vi "HFRR ADV v019 new software.vi"() -> ()   [LabVIEW 2025] (continued)
          tunnel: [w1633 w1647] -> w1619
          tunnel: w1611 -> [w1632 w1651]
          frame No Error {
            n1452 = property class="Instr"(reference=w1632, error in=w1631) -> (reference out=w1629:refnum<visa-resource-name>, error out=w1630:errorcluster, "Serial Settings:Number of Bytes at Serial Port"=w1626:u32)
            n1453 = Greater?(x=w1626, y=u32 5) -> (0:w1625:bool)
            n1454 = Not(x=w1625) -> (.not. x?=→"Port 1a":bool)
            n1455 = while {
              tunnel: [w1642] -> w1633
              tunnel: [w1641] -> w1634
              tunnel: w1630 -> [w1640]
              tunnel: w1629 -> [w1639]
              stop <- TRUE stop-if-true
              n1456 = property class="Instr" props=["Serial Settings:Number of Bytes at Serial Port"](reference=w1639, error in=w1640) -> (reference out=w1644:refnum<visa-resource-name>, error out=w1643:errorcluster)  [unwired: 1 out]
              n1457 = VISA Read(VISA resource name=w1644, byte count=u32 50, error in (no error)=w1643) -> (VISA resource name out=w1641:refnum<visa-resource-name>, read buffer=→"UNI READ":string, error out=w1642:errorcluster)  [unwired: 1 out]
              n1458 = Wait (ms)(milliseconds to wait=u32 5) -> ()  [unwired: 1 out]
            }
          }
          frame Error {
            w1659 = u16 0 items=["None", "XON/XOFF", "RTS/CTS", "XON/XOFF & RTS/CTS", "DTR/DSR", "XON/XOFF & DTR/DSR"] ("flow control (0:none)  2")
            w1657 = u16 10 items=["1.0"=10, "1.5"=15, "2.0"=20] ("stop bits 2")
            w1655 = u16 0 items=["None", "Odd", "Even", "Mark", "Space"] ("parity 2")
            w1656 = u32 10000  # timeout (10sec)
            n1459 = VISA Close(VISA resource name=w1651, error in (no error)=w1649) -> (error out=w1652:errorcluster)
            n1460 = local write "Port 1a"(FALSE ("Port 1a")) -> ()
            n1461 = local read "Com Port 1"() -> (w1646:refnum<visa-resource-name>)
            n1462 = call <vilib>:"Clear Errors.vi"("error in (no error)"=w1652) -> ("error out"=w1650:errorcluster)  [unwired: 5 in, 1 out]
            n1463 = call-poly "VISA Configure Serial Port"("VISA resource name"=w1646, "timeout (10sec)"=w1656, "baud rate (9600)"=u32 250000 ("baud rate  2"), "data bits (8)"=u16 8 ("data bits  2"), "parity (0:none)"=w1655, "error in (no error)"=w1650, "stop bits (10: 1 bit)"=w1657, "flow control (0:none)"=w1659) -> ("VISA resource name out"=w1660:refnum<visa-resource-name>, "error out"=w1661:errorcluster)  [unwired: 6 in]
            n1464 = flat-sequence {
              tunnel: w1660 -> [w1663]
              tunnel: w1661 -> [w1662]
              tunnel: [w1663] -> w1653
              tunnel: [w1662] -> w1647
              frame #0 {
                n1465 = Wait (ms)(milliseconds to wait=u32 50) -> ()  [unwired: 1 out]
              }
            }
            "Residual Uno" <- ""
            "Port 1 Error" <- w1647
          }
        }
        n1466 = local read "Quit"() -> (w1608:bool)
        "Error Uno" <- w1613
      }
      n1467 = VISA Close(VISA resource name=w1606, error in (no error)=w1605) -> (error out=w1603:errorcluster)
      n1468 = call <vilib>:"Clear Errors.vi"("error in (no error)"=w1603) -> ()  [unwired: 5 in, 2 out]
    }
    frame Enabled {
    }
  }
  n1469 = while {
    stop <- w1674 stop-if-true
    # "V0OLTAGE TO STROKE (peice vise calibration)"
    n1470 = local read "LVDT MIN"() -> (w1665:dbl)
    n1471 = Wait (ms)(milliseconds to wait=u32 10) -> ()  [unwired: 1 out]
    n1472 = local read "LVDT Peak"() -> (w1666:dbl)
    n1473 = formula code="// Dynamic Parameterized Linear Interpolation Node\n// Inputs: vpp_val, voltages (Array), distances (Array)\n// Outputs: stroke\n\nint i = 0;\nint segments = 11; // 12 points make 11 interpolation segments\n\n// 1. Lower Boundary Clamp\nif (vpp_val <= voltages[0]) {\n    stroke = distances[0];\n}\n// 2. Upper Boundary Clamp\nelse if (vpp_val >= voltages[segments]) {\n    stroke = distances[segments];\n}\n// 3. Dynamic Segment Search Loop\nelse {\n    stroke = distances[0]; // Fallback baseline\n    for (i = 0; i < segments; i++) {\n        if (vpp_val >= voltages[i] && vpp_val <= voltages[i+1]) {\n            // Standard linear interpolation formula using array lookups\n            stroke = distances[i] + (vpp_val - voltages[i]) * (distances[i+1] - distances[i]) / (voltages[i+1] - voltages[i]);\n            break; // Segment found, safely exit the loop\n        }\n    }\n}"("vpp_val"=w1666, "voltages"="calibration values", "distances"="STROKE") -> ("stroke"=→"LVDT STROKE":dbl)
    n1474 = local read "Calibration Tare Value"() -> (w1670:dbl)
    n1475 = local read "Calibration Tare"() -> (w1668:bool)
    n1476 = Subtract(x=w1665, y=w1670) -> (x-y=→"LVDT STROKE  Calibration":dbl)
    n1477 = case shown="True" w1668 {
      selector: w1668 -> [_ w1676]
      tunnel: w1665 -> [_ w1677]
      frame False {
      }
      frame True {
        n1478 = Not(x=w1676) -> (.not. x?=w1675:bool)
        n1479 = local write "Calibration Tare"(w1675) -> ()
        "Calibration Tare Value" <- w1677
      }
    }
    n1480 = local read "Quit"() -> (w1674:bool)
  }
  n1481 = while {
    stop <- w1697 stop-if-true
    n1482 = call <vilib>:"High Resolution Polling Wait.vi"("seconds to wait"=0.02) -> ()  [unwired: 10 in, 1 out]
    n1483 = local read "Due read"() -> (w1695:string)
    n1484 = Spreadsheet String To Array(delimiter (Tab)=";", format string="", spreadsheet string=w1695, array type (2D Dbl)=string[] []) -> (array=w1692:string[])
    n1485 = Fract/Exp String To Number(string=w1692) -> (number=w1691:dbl[])  [unwired: 3 in, 1 out]
    n1486 = Index Array(array=w1691) -> (element #1=→"Sample Temperature":dbl, element #2=→"Target Sample Temperature":dbl, element #3=→"Current Duty Cycle":dbl, element #4=→"Ambient Temperature":dbl, element #5=→"Dac Status":dbl, element #6=→"Vpp":dbl, element #7=→"Active Error Code":dbl, element #8=→"Kp":dbl, element #9=→"Ki":dbl, element #10=→"Kd":dbl, element #11=→"SampleRaw":dbl, element #12=→"AmbRaw":dbl)  [unwired: 12 in]
    n1487 = local read "Quit"() -> (w1697:bool)
  }
  n1488 = while {
    shift-right: [w1711] -> w39
    shift-left: _ -> [w1702]
    shift-right: [w1710] -> w38
    shift-left: errorcluster {"status"=FALSE, "code"=0, "source"="Init"} ("error out") -> [w1704]
    tunnel: [w1699] -> w43
    tunnel: [w1709] -> _
    i -> [w1709]
    stop <- w1699 stop-if-true
    n1489 = local read "Com Port 2"() -> (w1703:refnum<visa-resource-name>)
    n1490 = local read "Port 2a"() -> (w1705:bool)
    n1491 = Unbundle(w1704) -> ("status"=→"Port 4":bool)  [unwired: 2 out]
    n1492 = call <vilib>:"High Resolution Polling Wait.vi"("seconds to wait"=0.02) -> ()  [unwired: 10 in, 1 out]
    n1493 = local read "Port 4"() -> (w1706:bool)
    n1494 = Not Equal?(x=w1703, y=w1702) -> (x != y?=w1701:bool)
    n1495 = Or(x=w1706, y=w1705) -> (x .or. y?=w1708:bool)
    n1496 = case shown="False" w1708 {
      frame False {
        w1714 = TRUE ("Visible")
        n1497 = property on="Port 2a" class="Bool (strict)"("Visible"=w1714) -> ()  [unwired: 2 in, 2 out]
        n1498 = property on="Port 4" class="Bool (strict)"("Visible"=w1714) -> ()  [unwired: 2 in, 2 out]
      }
      frame True {
        w1715 = TRUE ("Visible")
        n1499 = property on="Port 2a" class="Bool (strict)"("Visible"=w1715) -> ()  [unwired: 2 in, 2 out]
        n1500 = property on="Port 4" class="Bool (strict)"("Visible"=w1715) -> ()  [unwired: 2 in, 2 out]
      }
    }
    n1501 = case shown="True" w1701 {
      tunnel: [w1712 errorcluster {"status"=TRUE, "code"=0, "source"="Init"} ("error out")] -> w1700
      tunnel: w1704 -> [w1712 _]
      frame False {
      }
      frame True {
      }
    }
    n1502 = case shown="No Error" w1700 {
      selector: w1700 -> [w1728 w1759]
      tunnel: [w1721 w1764] -> w1711
      tunnel: [w1729 w1757] -> w1710
      tunnel: w1702 -> [w1730 w1762]
      frame No Error {
        n1503 = property class="Instr" props=["Serial Settings:Number of Bytes at Serial Port"](reference=w1730, error in=w1728) -> (reference out=w1722:refnum<visa-resource-name>, error out=w1727:errorcluster)  [unwired: 1 out]
        n1504 = while {
          tunnel: [w1738] -> w1723
          tunnel: [w1737] -> w1724
          tunnel: w1727 -> [w1736]
          tunnel: w1722 -> [w1735]
          tunnel: [w1734] -> _
          i -> [w1734]
          stop <- TRUE stop-if-true
          n1505 = property class="Instr" props=["Serial Settings:Number of Bytes at Serial Port"](reference=w1735, error in=w1736) -> (reference out=w1740:refnum<visa-resource-name>, error out=w1739:errorcluster)  [unwired: 1 out]
          n1506 = VISA Read(VISA resource name=w1740, byte count=u32 1000, error in (no error)=w1739) -> (VISA resource name out=w1737:refnum<visa-resource-name>, read buffer=→"Due read":string, error out=w1738:errorcluster)  [unwired: 1 out]
        }
        n1507 = local read "Command"() -> (w1720:string)
        n1508 = call <vilib>:"Trim Whitespace.vi"("string"=w1720) -> ("trimmed string"=w1719:string)  [unwired: 1 in]
        n1509 = Not Equal?(x=w1719, y="") -> (x != y?=w1725:bool)
        n1510 = VISA Flush I/O Buffer(VISA resource name=w1724) -> (VISA resource name out=w1717:refnum<visa-resource-name>, error out=→"error out 10":errorcluster)  [unwired: 2 in]
        n1511 = case shown="True" w1725 {
          tunnel: w1717 -> [w1742 w1747]
          tunnel: [w1742 w1751] -> w1721
          tunnel: w1723 -> [w1741 w1746]
          tunnel: [w1741 w1749] -> w1729
          tunnel: w1719 -> [_ w1745]
          tunnel: [_ w1748] -> _
          frame False {
            # "DATA  WRITE LOOP"
          }
          frame True {
            n1512 = Concatenate Strings(w1745, "\r\n") -> (w1744:string)
            n1513 = VISA Write(VISA resource name=w1747, write buffer=w1744, error in (no error)=w1746) -> (VISA resource name out=w1751:refnum<visa-resource-name>, return count=w1748:u32, error out=w1750:errorcluster)
            n1514 = flat-sequence {
              tunnel: w1750 -> [w1753]
              tunnel: [w1753] -> w1749
              frame #0 {
                n1515 = local write "Command"("" ("Command")) -> ()
                n1516 = Wait (ms)(milliseconds to wait=u32 5) -> ()  [unwired: 1 out]
              }
            }
          }
        }
        "Port 2a" <- TRUE ("Port 2a")
      }
      frame Error {
        w1770 = u16 0 items=["None", "XON/XOFF", "RTS/CTS", "XON/XOFF & RTS/CTS", "DTR/DSR", "XON/XOFF & DTR/DSR"] ("flow control (0:none)  2")
        w1768 = u16 10 items=["1.0"=10, "1.5"=15, "2.0"=20] ("stop bits 2")
        w1766 = u16 0 items=["None", "Odd", "Even", "Mark", "Space"] ("parity 2")
        w1767 = u32 10000  # timeout (10sec)
        n1517 = VISA Clear(VISA resource name=w1762, error in (no error)=w1759) -> (VISA resource name out=w1761:refnum<visa-resource-name>, error out=w1760:errorcluster)
        n1518 = VISA Close(VISA resource name=w1761, error in (no error)=w1760) -> (error out=w1763:errorcluster)
        n1519 = call <vilib>:"Clear Errors.vi"("error in (no error)"=w1763) -> ()  [unwired: 5 in, 2 out]
        n1520 = local write "Port 2a"(FALSE ("Port 2a")) -> ()
        n1521 = local read "Com Port 2"() -> (w1756:refnum<visa-resource-name>)
        "visa due" <- w1756
        n1522 = call-poly "VISA Configure Serial Port"("VISA resource name"=w1756, "timeout (10sec)"=w1767, "baud rate (9600)"=u32 250000 ("baud rate  2"), "data bits (8)"=u16 8 ("data bits  2"), "parity (0:none)"=w1766, "stop bits (10: 1 bit)"=w1768, "flow control (0:none)"=w1770) -> ("VISA resource name out"=w1771:refnum<visa-resource-name>, "error out"=w1772:errorcluster)  [unwired: 7 in]
        n1523 = flat-sequence {
          tunnel: w1771 -> [w1774]
          tunnel: w1772 -> [w1773]
          tunnel: [w1774] -> w1764
          tunnel: [w1773] -> w1757
          frame #0 {
            n1524 = Wait (ms)(milliseconds to wait=u32 50) -> ()  [unwired: 1 out]
          }
        }
        "Residual Due" <- ""
        "Port 2 Error" <- w1757
      }
    }
    n1525 = local read "Quit"() -> (w1699:bool)
    "Error Due" <- w1704
  }
  n1526 = local write "FRICVALZ"(0.0 ("FRICVALZ")) -> ()
  n1527 = property on="RUN" class="Bool (strict)"("Visible"=TRUE) -> ()  [unwired: 2 in, 2 out]
  n1528 = while {
    tunnel: [w1791] -> _
    tunnel: [w1776] -> w53
    i -> [w1791]
    stop <- w1776 stop-if-true
    n1529 = local read "conststatus"() -> (w1780:dbl)
    n1530 = local read "Main Tab"() -> (w1778:T2)
    n1531 = local read "EDIT"() -> (w1797:bool)
    n1532 = local read "Rate"() -> (w1796:dbl)
    n1533 = case shown="True" w1797 {
      tunnel: [FALSE TRUE] -> w1783
      frame False {
      }
      frame True {
      }
    }
    n1534 = property on="Time slide" class="Slide (strict)"("Scale.Range:Maximum"=2500.0) -> ()  [unwired: 2 in, 2 out]
    n1535 = Equal?(x=w1778, y=T27."About" ("Main Tab")) -> (x = y?=w1789:bool)
    n1536 = Equal?(x=w1780, y=0.0) -> (x = y?=w1781:bool)
    n1537 = Divide(x=1.0, y=w1796) -> (x/y=w1792:dbl)
    "Time 2" <- w1792
    n1538 = case shown="True" w1781 {
      frame False {
      }
      frame True {
        # "C:\\WinDucom\\calibrate WO 2391.dcf"
        n1539 = local write "Lan flag"(22) -> ()
        n1540 = local write "conststatus"(10.0 ("rpm value : 2")) -> ()
        n1541 = String To Path(string="C:\\LAB-IQ\\calibrate WO 2465.dcf") -> (path=w1803:path)
        n1542 = Open/Create/Replace File "Open File"(file path (use dialog)=w1803) -> (refnum out=w1801:refnum<file>)  [unwired: 5 in, 2 out]
        n1543 = for {
          N: 23 -> [_]
          tunnel: w1801 -> [w1812]
          i -> [w1806]
          (unwired) TRUE ("line mode (F)")
          n1544 = Read from Text File "Read File"(file (use dialog)=w1812) -> (text=w1811:string)  [unwired: 3 in, 3 out]
          n1545 = Match Pattern(string=w1811, regular expression="]") -> (after substring=w1809:string)  [unwired: 1 in, 3 out]
          n1546 = String Subset(string=w1811, offset (0)=5, length (rest)=10 ("length (rest)")) -> (substring=w1804:string)
          n1547 = Fract/Exp String To Number(string=w1804) -> (number=w1805:dbl)  [unwired: 3 in, 1 out]
          n1548 = Match Pattern(string=w1809, regular expression="-") -> (before substring=w1807:string)  [unwired: 1 in, 3 out]
          n1549 = case shown="4" w1806 {
            tunnel: w1805 -> [w1815 w1816 w1817 w1818 _ _ _ w1823 w1824 _ w1825 w1826 w1827 w1828 w1829 w1830 _ w1831 w1832 _ _ _ _ _]
            tunnel: w1807 -> [_ _ _ _ w1819 w1820 w1821 _ _ _ _ _ _ _ _ _ _ _ _ w1833 w1834 w1835 w1836 _]
            frame 0 {
              n1550 = local write "FRIC. FORCE :"(w1815) -> ()
            }
            frame 1 {
              n1551 = local write "TEMPERATURE :"(w1816) -> ()
            }
            frame 2 {
              n1552 = local write "HUMIDITY:"(w1817) -> ()
            }
            frame 3 {
              n1553 = local write "AIR TEMPERATURE :"(w1818) -> ()
            }
            frame 4 {
              n1554 = local write "Com Port 1"(w1819) -> ()
            }
            frame 5 {
              n1555 = local write "Com Port 2"(w1820) -> ()
              n1556 = local write "visa due"(w1820) -> ()
            }
            frame 6 {
              n1557 = String To Path(string=w1821) -> (path=w1822:path)
              n1558 = local write "File Path"(w1822) -> ()
              "String" <- w1821
            }
            frame 7 {
              n1559 = local write "DISPLACEMENT :"(w1823) -> ()
            }
            frame 8 {
              n1560 = local write "STROKE GAIN :"(w1824) -> ()
            }
            frame 9 {
            }
            frame 10 {
              n1561 = local write "Language Selection"(w1825) -> ()
            }
            frame 11 {
              n1562 = local write "CH-POWER +"(w1826) -> ()
            }
            frame 12 {
              n1563 = local write "CH-POWER -"(w1827) -> ()
            }
            frame 13 {
              n1564 = local write "CH-HEATER"(w1828) -> ()
            }
            frame 14 {
              n1565 = local write "CH-HUMIDITY WET"(w1829) -> ()
            }
            frame 15 {
              n1566 = local write "CH-HUMIDITY DRY"(w1830) -> ()
            }
            frame 16 {
            }
            frame 17 {
              n1567 = local write "AIR TEMP INTERCEPT:"(w1831) -> ()
            }
            frame 18 {
              n1568 = local write "TEMP INTERCEPT:"(w1832) -> ()
            }
            frame 21 {
              n1569 = local write "S.NO"(w1833) -> ()
            }
            frame 22 {
              n1570 = local write "Com Port 3"(w1834) -> ()
            }
            frame 20 {
              n1571 = local write "Camera Port :"(w1835) -> ()
            }
            frame 19 {
              n1572 = local write "C3 :"(w1836) -> ()
            }
            frame 23, Default {
            }
          }
        }
      }
    }
    n1573 = Select(t=u32 2500 ("milliseconds to wait"), s=w1789, f=u32 500 ("milliseconds to wait")) -> (s? t:f=w1787:u32)
    n1574 = Multiply(x=w1792, y=w1787) -> (x*y=w1794:dbl)
    n1575 = property on="Time slide" class="Slide (strict)"("Visible"=w1783) -> ()  [unwired: 2 in, 2 out]
    n1576 = call "Elapsed Time2"("Time Target (s)"=w1794, "Auto Reset"=TRUE) -> ("Time has Elapsed"=w1784:bool)  [unwired: 10 in, 7 out]
    n1577 = case shown="True" w1784 {
      frame False {
      }
      frame True {
        n1578 = stacked-sequence {
          frame #0 {
            # "DATA PROCESSING"
            # "115 mV/N"
            n1579 = local read "Sample Temperature"() -> (w1839:dbl)
            n1580 = local read "RH Numeric:"() -> (w1846:dbl)
            n1581 = local read "HUMIDITY:"() -> (w1847:dbl)
            n1582 = local read "FRICVALZ"() -> (w1858:dbl)
            n1583 = local read "Friction"() -> (w1842:dbl)
            n1584 = Multiply(x=w1846, y=w1847) -> (x*y=→"Humidity ( %RH )" →"Hum" →"Hum 2":dbl)
            n1585 = call <vilib>:"Mean PtByPt.vi"("x"=w1839, "sample length"=100) -> ("mean"=w1838:dbl)  [unwired: 2 in, 1 out]
            "TEMP 2" <- w1838
            "TEMP 3" <- w1838
            n1586 = Subtract(x=w1842, y=w1858) -> (x-y=w1853:dbl)
            "FF 2" <- w1853
            "FF 4" <- w1853
            n1587 = local read "Ambient Temperature"() -> (→"AIR TEMP":dbl)
            n1588 = local read "TEMP"() -> (w1857:dbl)
            n1589 = local write "FF 3"(w1853) -> ()
            n1590 = Compound Arithmetic op=OR("FRICVALZ 4", "FRICVALZ 3", "FRICVALZ 2") -> (w1849:bool)
            n1591 = case shown="True" w1849 {
              tunnel: w1842 -> [_ w1864]
              frame False {
              }
              frame True {
                w1863 = FALSE ("FRICVALZ")
                n1592 = local write "FRICVALZ 3"(w1863) -> ()
                n1593 = local write "FRICVALZ 2"(w1863) -> ()
                n1594 = local write "FRICVALZ 4"(w1863) -> ()
                "FRICVALZ" <- w1864
              }
            }
            n1595 = Not A Number/Path/Refnum?(number/path/refnum=w1857) -> (NaN/Path/Refnum?=w1856:bool)
            n1596 = Not A Number/Path/Refnum?(number/path/refnum=w1853) -> (NaN/Path/Refnum?=w1855:bool)
            n1597 = Divide(x=w1853, y=1.96) -> (x/y=w1850:dbl)
            n1598 = Compound Arithmetic op=OR(w1856, w1855) -> (w1854:bool)
            n1599 = Not A Number/Path/Refnum?(number/path/refnum=w1850) -> (NaN/Path/Refnum?=w1851:bool)
            n1600 = case shown="True" w1854 {
              frame False {
              }
              frame True {
                n1601 = local write "TEMP"(0.0 ("TEMP")) -> ()
                n1602 = local write "FF 2"(0.0 ("FF 2")) -> ()
                n1603 = local write "reinit"(TRUE ("reinit")) -> ()
              }
            }
            n1604 = local write "TEMP"(w1838) -> ()
            n1605 = Select(t=0.0, s=w1851, f=w1850) -> (s? t:f=w1841:dbl)
            "COF 2" <- w1841
            n1606 = local write "COF 3"(w1841) -> ()
          }
        }
      }
    }
    n1607 = Wait (ms)(milliseconds to wait=u32 50) -> ()  [unwired: 1 out]
    n1608 = local read "Quit"() -> (w1776:bool)
    "Rate" <- 2500.0 ("No of Samples")
  }
  n1609 = while {
    tunnel: w56 -> [_]
    tunnel: [w1891] -> _
    tunnel: [w1867] -> w55
    i -> [w1891]
    stop <- w1867 stop-if-true
    # "C:\\LAB-IQ-NXT\\Scar View.exe"
    n1610 = local read "OK Button 16"() -> (w1880:bool)
    n1611 = local read "Main Tab"() -> (w1873:T2)
    n1612 = local read "service 3"() -> (w1874:bool)
    n1613 = local read "OPEN 6"() -> (w1876:bool)
    n1614 = local read "EDIT 2"() -> (w1878:bool)
    n1615 = flat-sequence {
      frame #0 {
        n1616 = local read "SAVE 2"() -> (w2493:bool)
        n1617 = stacked-sequence {
          frame #0 {
            n1618 = local read "EDIT"() -> (w2547:bool)
            n1619 = case shown="True" w2547 {
              tunnel: [u8 2 ("Disabled") u8 0 ("Disabled")] -> _
              frame False {
                w2549 = FALSE
                n1620 = local write "Password"("") -> ()
                n1621 = property on="SrvM CP" class="Bool (strict)"("Visible"=w2549) -> ()  [unwired: 2 in, 2 out]
                n1622 = property on="message" class="Str"("Visible"=w2549) -> ()  [unwired: 2 in, 2 out]
                n1623 = local write "x = y?"(w2549) -> ()
                n1624 = property on="Password" class="Str"("Visible"=w2549) -> ()  [unwired: 2 in, 2 out]
                n1625 = property on="ENTER THE NEW PASSWORD" class="Str"("Visible"=w2549) -> ()  [unwired: 2 in, 2 out]
                n1626 = property on="ENTER CURRENT PASSWORD" class="Str"("Visible"=w2549) -> ()  [unwired: 2 in, 2 out]
                n1627 = local write "SrvM CP"(w2549) -> ()
              }
              frame True {
                w2552 = TRUE
                n1628 = property on="SrvM CP" class="Bool (strict)"("Visible"=w2552) -> ()  [unwired: 2 in, 2 out]
                n1629 = property on="Password" class="Str"("Visible"=w2552) -> ()  [unwired: 2 in, 2 out]
              }
            }
            "dipl pwd" <- "@143$\n" ("dipl pwd")
          }
          frame #1 {
            # "Gain password"
            n1630 = String To Byte Array(string="ENTER CURRENT PASSWORD") -> (unsigned byte array=w2557:u8[])
            n1631 = Search 1D Array(1D array=w2557, element=u8 10) -> (index of element=w2560:i32)  [unwired: 1 in]
            n1632 = Index Array(array=w2557, index=w2560) -> (element=w2556:u8)
            n1633 = Equal?(x=w2556, y=10) -> (x = y?=w2554:bool)
            n1634 = case shown="True" w2554 {
              frame False {
                n1635 = property on="ENTER THE NEW PASSWORD" class="Str"("Visible"=FALSE) -> ()  [unwired: 2 in, 2 out]
              }
              frame True {
                # "password"
                # "change password logic"
                n1636 = local read "ENTER CURRENT PASSWORD"() -> (w2573:string)
                n1637 = local read "dipl pwd"() -> (w2567:string)
                n1638 = String To Byte Array(string=w2573) -> (unsigned byte array=w2575:u8[])
                n1639 = String To Byte Array(string=w2567) -> (unsigned byte array=w2568:u8[])
                n1640 = Array Size(array=w2575) -> (size(s)=w2572:i32)
                n1641 = Array Size(array=w2568) -> (size(s)=w2570:i32)
                n1642 = for {
                  N: w2572 -> [_]
                  tunnel: w2575 -> [w2599]
                  tunnel: [w2597] -> w2576 mode=indexing
                  tunnel: w2572 -> [w2591]
                  i -> [w2592]
                  n1643 = Decrement(x=w2591) -> (x-1=w2589:i32)
                  n1644 = Equal?(x=w2592, y=w2589) -> (x = y?=w2590:bool)
                  n1645 = Index Array(array=w2599, index=w2592) -> (element=w2593:u8)
                  n1646 = Number To Decimal String(number=w2593) -> (decimal integer string=w2598:string)  [unwired: 1 in]
                  n1647 = Select(t="", s=w2590, f="\r") -> (s? t:f=w2595:string)
                  n1648 = Concatenate Strings(w2598, w2595) -> (w2597:string)
                }
                n1649 = for {
                  N: w2570 -> [_]
                  tunnel: w2568 -> [w2587]
                  tunnel: [w2585] -> w2569 mode=indexing
                  tunnel: w2570 -> [w2582]
                  i -> [w2583]
                  n1650 = Decrement(x=w2582) -> (x-1=w2581:i32)
                  n1651 = Equal?(x=w2583, y=w2581) -> (x = y?=w2580:bool)
                  n1652 = Index Array(array=w2587, index=w2583) -> (element=w2586:u8)
                  n1653 = Number To Decimal String(number=w2586) -> (decimal integer string=w2584:string)  [unwired: 1 in]
                  n1654 = Select(t="", s=w2580, f="\r") -> (s? t:f=w2577:string)
                  n1655 = Concatenate Strings(w2584, w2577) -> (w2585:string)
                }
                n1656 = local read "string"() -> (w2574:string)
                n1657 = Concatenate Strings(w2569) -> (w2563:string)
                n1658 = Concatenate Strings(w2574) -> (w2571:string)
                n1659 = Concatenate Strings(w2576) -> (w2564:string)
                n1660 = Equal?(x=w2564, y=w2571) -> (x = y?=w2566:bool)
                n1661 = Equal?(x=w2564, y=w2563) -> (x = y?=w2562:bool)
                n1662 = Or(x=w2566, y=w2562) -> (x .or. y?=w2565:bool)
                n1663 = case shown="True" w2565 {
                  frame False {
                  }
                  frame True {
                    n1664 = property on="ENTER THE NEW PASSWORD" class="Str"("Visible"=TRUE) -> ()  [unwired: 2 in, 2 out]
                  }
                }
              }
            }
          }
          frame #2 {
            n1665 = String To Byte Array(string="ENTER THE NEW PASSWORD") -> (unsigned byte array=w2602:u8[])
            n1666 = Search 1D Array(1D array=w2602, element=u8 10) -> (index of element=w2606:i32)  [unwired: 1 in]
            n1667 = Index Array(array=w2602, index=w2606) -> (element=w2604:u8)
            n1668 = Equal?(x=w2604, y=10) -> (x = y?=w2601:bool)
            n1669 = case shown="False" w2601 {
              frame False {
              }
              frame True {
                n1670 = local write "EDIT"(FALSE) -> ()
                n1671 = local write "SrvM CP"(FALSE) -> ()
                n1672 = local read "ENTER THE NEW PASSWORD"() -> (w2609:string)
                n1673 = String To Byte Array(string=w2609) -> (unsigned byte array=w2614:u8[])
                n1674 = Array Size(array=w2614) -> (size(s)=w2611:i32)
                n1675 = for {
                  N: w2611 -> [_]
                  tunnel: w2614 -> [w2627]
                  tunnel: [w2624] -> w2616 mode=indexing
                  tunnel: w2611 -> [w2619]
                  i -> [w2617]
                  n1676 = Decrement(x=w2619) -> (x-1=w2620:i32)
                  n1677 = Equal?(x=w2617, y=w2620) -> (x = y?=w2621:bool)
                  n1678 = Index Array(array=w2627, index=w2617) -> (element=w2626:u8)
                  n1679 = Number To Decimal String(number=w2626) -> (decimal integer string=w2625:string)  [unwired: 1 in]
                  n1680 = Select(t="", s=w2621, f="\r") -> (s? t:f=w2618:string)
                  n1681 = Concatenate Strings(w2625, w2618) -> (w2624:string)
                }
                n1682 = local read "file path"() -> (w2608:path)
                n1683 = Concatenate Strings(w2616) -> (w2610:string)
                n1684 = Delete(path (use dialog)=w2608) -> (deleted path=w2612:path)  [unwired: 4 in, 2 out]
                n1685 = call <vilib>:"Write Characters To File.vi"("append to file? (new file:F)"=FALSE, "character string"=w2610, "file path (dialog if empty)"=w2612) -> ()  [unwired: 2 in, 1 out]
              }
            }
          }
          frame #3 {
            n1686 = case shown="True" "SrvM CP" {
              frame False {
                w2630 = ""
                n1687 = local write "ENTER CURRENT PASSWORD"(w2630) -> ()
                n1688 = local write "ENTER THE NEW PASSWORD"(w2630) -> ()
                n1689 = property on="ENTER CURRENT PASSWORD" class="Str"("Visible"=FALSE) -> ()  [unwired: 2 in, 2 out]
              }
              frame True {
                n1690 = property on="ENTER THE NEW PASSWORD" class="Str"() -> ("Visible"=w2631:bool)  [unwired: 2 in, 2 out]
                n1691 = Not(x=w2631) -> (.not. x?=w2632:bool)
                n1692 = property on="ENTER CURRENT PASSWORD" class="Str"("Visible"=w2632) -> ()  [unwired: 2 in, 2 out]
              }
            }
          }
          frame #4 {
            n1693 = String To Byte Array(string="Password") -> (unsigned byte array=w2639:u8[])
            n1694 = Search 1D Array(1D array=w2639, element=u8 10) -> (index of element=w2637:i32)  [unwired: 1 in]
            n1695 = Index Array(array=w2639, index=w2637) -> (element=w2638:u8)
            n1696 = Equal?(x=w2638, y=10) -> (x = y?=w2634:bool)
            n1697 = case shown="True" w2634 {
              frame False {
              }
              frame True {
                # "password"
                # "password"
                n1698 = local read "Password"() -> (w2652:string)
                n1699 = String To Byte Array(string=w2652) -> (unsigned byte array=w2655:u8[])
                n1700 = String To Byte Array(string="@143$\n") -> (unsigned byte array=w2641:u8[])
                n1701 = Array Size(array=w2655) -> (size(s)=w2650:i32)
                n1702 = Array Size(array=w2641) -> (size(s)=w2646:i32)
                n1703 = for {
                  N: w2650 -> [_]
                  tunnel: w2655 -> [w2689]
                  tunnel: [w2687] -> w2656 mode=indexing
                  tunnel: w2650 -> [w2684]
                  i -> [w2685]
                  n1704 = Decrement(x=w2684) -> (x-1=w2683:i32)
                  n1705 = Index Array(array=w2689, index=w2685) -> (element=w2688:u8)
                  n1706 = Equal?(x=w2685, y=w2683) -> (x = y?=w2682:bool)
                  n1707 = Number To Decimal String(number=w2688) -> (decimal integer string=w2686:string)  [unwired: 1 in]
                  n1708 = Select(t="", s=w2682, f="\r") -> (s? t:f=w2679:string)
                  n1709 = Concatenate Strings(w2686, w2679) -> (w2687:string)
                }
                n1710 = for {
                  N: w2646 -> [_]
                  tunnel: w2641 -> [w2700]
                  tunnel: [w2698] -> w2644 mode=indexing
                  tunnel: w2646 -> [w2695]
                  i -> [w2696]
                  n1711 = Decrement(x=w2695) -> (x-1=w2694:i32)
                  n1712 = Index Array(array=w2700, index=w2696) -> (element=w2699:u8)
                  n1713 = Equal?(x=w2696, y=w2694) -> (x = y?=w2693:bool)
                  n1714 = Number To Decimal String(number=w2699) -> (decimal integer string=w2697:string)  [unwired: 1 in]
                  n1715 = Select(t="", s=w2693, f="\r") -> (s? t:f=w2690:string)
                  n1716 = Concatenate Strings(w2697, w2690) -> (w2698:string)
                }
                n1717 = local read "file path"() -> (w2640:path)
                n1718 = call <vilib>:"Read Characters From File.vi"("file path (dialog if empty)"=w2640) -> ("character string"=w2654:string)  [unwired: 5 in, 3 out]
                "string" <- w2654
                n1719 = flat-sequence {
                  tunnel: [w2657] -> w2651
                  frame #0 {
                    w2657 = ""
                    n1720 = local write "Password"(w2657) -> ()
                  }
                }
                n1721 = Concatenate Strings(w2644) -> (w2645:string)
                n1722 = Concatenate Strings(w2654) -> (w2653:string)
                n1723 = Concatenate Strings(w2656) -> (w2648:string)
                n1724 = Equal?(x=w2648, y=w2653) -> (x = y?=w2643:bool)
                n1725 = Equal?(x=w2648, y=w2645) -> (x = y?=w2649:bool)
                n1726 = Or(x=w2643, y=w2649) -> (x .or. y?=w2642:bool)
                "x = y?" <- w2642
                n1727 = case shown="True" w2642 {
                  selector: w2642 -> [w2659 _]
                  tunnel: w2651 -> [_ _]
                  frame False {
                    n1728 = And(x=w2659, y=TRUE ("Visible")) -> (x .and. y?=w2660:bool)
                    n1729 = property on="message" class="Str"("Visible"=w2660) -> ()  [unwired: 2 in, 2 out]
                  }
                  frame True {
                    n1730 = control-ref of="This VI"() -> (w2671:refnum<vi>)
                    n1731 = property class="VI"(reference=w2671) -> (reference out=w2662:refnum<vi>, error out=w2666:errorcluster, "Panel"=w2670:refnum<vi>)  [unwired: 1 in]
                    n1732 = property on="message" class="Str"("Visible"=FALSE) -> ()  [unwired: 2 in, 2 out]
                    n1733 = property class="Pnl"(reference=w2670, error in=w2666) -> (reference out=w2664:refnum<vi>, error out=w2667:errorcluster, "Panes[]"=w2669:refnum<vi>[])
                    n1734 = for {
                      tunnel: w2669 -> [w2678] mode=indexing
                      tunnel: T21."Always On" ("Horizontal Scrollbar Visibility") -> [w2677]
                      tunnel: w2667 -> [w2674]
                      tunnel: [w2673] -> w2665
                      n1735 = property class="Pane"(reference=w2678, error in=w2674, "HorizScrollbarVisibility"=w2677) -> (reference out=w2675:refnum<vi>, error out=w2676:errorcluster)
                      n1736 = Close Reference(reference=w2675, error in (no error)=w2676) -> (error out=w2673:errorcluster)
                    }
                    n1737 = Close Reference(reference=w2664, error in (no error)=w2665) -> (error out=w2663:errorcluster)
                    n1738 = Close Reference(reference=w2662, error in (no error)=w2663) -> (error out=→"error out 6":errorcluster)
                  }
                }
              }
            }
          }
        }
        n1739 = local read "x = y?"() -> (w2499:bool)
        n1740 = local read "HUMIDITY: 2"() -> (w2501:dbl)
        n1741 = local read "HUMIDITY:"() -> (w2500:dbl)
        n1742 = property on="Port 2 Error" class="Clust (strict)"("Visible"="EDIT") -> ()  [unwired: 2 in, 2 out]
        n1743 = property on="Port 1 Error" class="Clust (strict)"("Visible"="EDIT") -> ()  [unwired: 2 in, 2 out]
        n1744 = case shown="True" "SrvM CP 2" {
          frame False {
          }
          frame True {
            n1745 = local write "SrvM CP 2"(FALSE ("SrvM CP 2")) -> ()
            n1746 = local read "HUMIDITY: 2"() -> (w2540:dbl)
            n1747 = local read "TEMP INTERCEPT: 2"() -> (w2539:dbl)
            n1748 = local read "DISPLACEMENT : 4"() -> (w2543:dbl)
            n1749 = local read "TEMPERATURE : 2"() -> (w2542:dbl)
            n1750 = local read "STROKE GAIN : 2"() -> (w2544:dbl)
            n1751 = local read "FRIC. FORCE : 2"() -> (w2545:dbl)
            n1752 = local read "AIR TEMP INTERCEPT: 2"() -> (w2538:dbl)
            n1753 = local read "AIR TEMPERATURE : 2"() -> (w2541:dbl)
            n1754 = local write "HUMIDITY:"(w2540) -> ()
            n1755 = local write "AIR TEMP INTERCEPT:"(w2539) -> ()
            n1756 = local write "TEMPERATURE :"(w2542) -> ()
            n1757 = local write "FRIC. FORCE :"(w2545) -> ()
            n1758 = local write "STROKE GAIN :"(w2544) -> ()
            n1759 = local write "DISPLACEMENT :"(w2543) -> ()
            n1760 = local write "AIR TEMPERATURE :"(w2541) -> ()
            n1761 = local write "TEMP INTERCEPT:"(w2538) -> ()
          }
        }
        n1762 = Or(x="SAVE", y=w2493) -> (x .or. y?=w2494:bool)
        n1763 = And(x="EDIT", y=w2499) -> (x .and. y?=w2497:bool)
        n1764 = local read "DISPLACEMENT : 4"() -> (w2510:dbl)
        n1765 = local read "TEMPERATURE : 2"() -> (w2508:dbl)
        n1766 = local read "STROKE GAIN : 2"() -> (w2514:dbl)
        n1767 = local read "DISPLACEMENT :"() -> (w2509:dbl)
        n1768 = local read "FRIC. FORCE : 2"() -> (w2517:dbl)
        n1769 = local read "TEMPERATURE :"() -> (w2506:dbl)
        n1770 = local read "STROKE GAIN :"() -> (w2513:dbl)
        n1771 = local read "FRIC. FORCE :"() -> (w2516:dbl)
        n1772 = case shown="True" w2497 {
          tunnel: [u8 2 ("Disabled") u8 0 ("Disabled")] -> w2496
          tunnel: [w2861 TRUE ("Visible")] -> w2495
          frame False {
            w2861 = FALSE ("Visible")
            n1773 = local write "EDIT 2"(w2861) -> ()
          }
          frame True {
          }
        }
        n1774 = case shown="True" w2494 {
          frame False {
          }
          frame True {
            n1775 = stacked-sequence {
              seq-local: [w2709 _ _] -> [_ w2856 _]
              frame #0 {
                (unwired) i16 5 ("precision (6)")
                # "[CH1]    - FF\n[CH2]   - TEMPERATURE\n[CH3]    - Humidity\n[CH4]    - AIR TEMP\n[CH5]\\- Visa Uno\n[CH6] \\- Visa Due\n[CH7]  \\- file path\n[CH8]   - Displacement Gain\n[CHA]   - Stroke Gain\n[CHB]   - Stroke PID Gain\n[CHC]   -Language Selection\n[CHD]   -Power +\n[CHE]   -Power_\n[CHF]   -Heater\n[CHG]   -Humidity Wet\n[CHH]   -Humidity Dry\n[CHI]   -Integral Time"
                n1776 = local read "Language Selection"() -> (w2757:enum16{"English", "Russian"})
                n1777 = local read "CH-HUMIDITY WET"() -> (w2715:u16)
                n1778 = local read "CH-HUMIDITY DRY"() -> (w2712:u16)
                n1779 = local read "STROKE GAIN :"() -> (w2701:dbl)
                n1780 = local read "CH-POWER +"() -> (w2724:u16)
                n1781 = local read "CH-POWER -"() -> (w2721:u16)
                n1782 = local read "CH-HEATER"() -> (w2718:u16)
                n1783 = local read "AIR TEMPERATURE :"() -> (w2704:dbl)
                n1784 = local read "DISPLACEMENT :"() -> (w2702:dbl)
                n1785 = local read "TEMPERATURE :"() -> (w2705:dbl)
                n1786 = local read "FRIC. FORCE :"() -> (w2706:dbl)
                n1787 = local read "HUMIDITY:"() -> (w2703:dbl)
                n1788 = Path To String(path="File Path") -> (string=w2773:string)
                n1789 = Number To Fractional String(number=w2701, width (-)=i16 10 ("precision (6)"), precision (6)=i16 5) -> (F-format string=w2764:string)  [unwired: 1 in]
                n1790 = Number To Fractional String(number=w2757, width (-)=i16 10 ("precision (6)"), precision (6)=i16 5) -> (F-format string=w2753:string)  [unwired: 1 in]
                n1791 = Number To Fractional String(number=w2724, width (-)=i16 10 ("precision (6)"), precision (6)=i16 5) -> (F-format string=w2747:string)  [unwired: 1 in]
                n1792 = Number To Fractional String(number=w2721, width (-)=i16 10 ("precision (6)"), precision (6)=i16 5) -> (F-format string=w2744:string)  [unwired: 1 in]
                n1793 = Number To Fractional String(number=w2718, width (-)=i16 10 ("precision (6)"), precision (6)=i16 5) -> (F-format string=w2739:string)  [unwired: 1 in]
                n1794 = Number To Fractional String(number=w2715, width (-)=i16 10 ("precision (6)"), precision (6)=i16 5) -> (F-format string=w2736:string)  [unwired: 1 in]
                n1795 = Number To Fractional String(number=w2712, width (-)=i16 10 ("precision (6)"), precision (6)=i16 5) -> (F-format string=w2731:string)  [unwired: 1 in]
                n1796 = local read "Com Port 1"() -> (w2708:refnum<visa-resource-name>)
                n1797 = local read "Com Port 2"() -> (w2707:refnum<visa-resource-name>)
                n1798 = Concatenate Strings(w2773, "\\" ("string")) -> (w2772:string)
                n1799 = Number To Fractional String(number=w2706, width (-)=i16 10 ("precision (6)"), precision (6)=i16 5) -> (F-format string=w2805:string)  [unwired: 1 in]
                n1800 = Number To Fractional String(number=w2705, width (-)=i16 10 ("precision (6)"), precision (6)=i16 5) -> (F-format string=w2804:string)  [unwired: 1 in]
                n1801 = Number To Fractional String(number=w2703, width (-)=i16 10 ("precision (6)"), precision (6)=i16 5) -> (F-format string=w2798:string)  [unwired: 1 in]
                n1802 = Number To Fractional String(number=w2704, width (-)=i16 10 ("precision (6)"), precision (6)=i16 5) -> (F-format string=w2792:string)  [unwired: 1 in]
                n1803 = Number To Fractional String(number=w2702, width (-)=i16 10 ("precision (6)"), precision (6)=i16 5) -> (F-format string=w2765:string)  [unwired: 1 in]
                n1804 = Concatenate Strings("[CHA]" ("string"), w2764, "- Stroke Gain" ("string"), "\r") -> (w2758:string)
                n1805 = Concatenate Strings("[CHC]" ("string"), w2753, "-Language Selection" ("string"), "\r") -> (w2750:string)
                n1806 = Concatenate Strings("[CHD]" ("string"), w2747, "-Power +" ("string"), "\r") -> (w2729:string)
                n1807 = Concatenate Strings("[CHG]" ("string"), w2736, "-Humidity Wet" ("string"), "\r") -> (w2726:string)
                n1808 = Concatenate Strings("[CHH]" ("string"), w2731, "-Humidity Dry" ("string"), "\r") -> (w2725:string)
                n1809 = Concatenate Strings("[CH1]" ("string"), w2805, " - FF" ("string"), "\r") -> (w2803:string)
                n1810 = Concatenate Strings("[CH2]" ("string"), w2804, " - TEMPERATURE" ("string"), "\r") -> (w2802:string)
                n1811 = Concatenate Strings("[CH3]" ("string"), w2798, " - Humidity" ("string"), "\r") -> (w2795:string)
                n1812 = Concatenate Strings("[CH4]" ("string"), w2792, " - AIR TEMP" ("string"), "\r") -> (w2788:string)
                n1813 = Concatenate Strings("[CH5]" ("string"), w2708, "- Visa Uno" ("string"), "\r") -> (w2781:string)
                n1814 = Concatenate Strings("[CH6]" ("string"), w2707, "- Visa Due" ("string"), "\r") -> (w2776:string)
                n1815 = Concatenate Strings("[CH7]" ("string"), w2772, "- file path" ("string"), "\r") -> (w2775:string)
                n1816 = Concatenate Strings("[CH8]" ("string"), w2765, "- Displacement Gain" ("string"), "\r") -> (w2768:string)
                n1817 = Concatenate Strings("[CHE]" ("string"), w2744, "-Power_" ("string"), "\r") -> (w2728:string)
                n1818 = Concatenate Strings("[CHF]" ("string"), w2739, "-Heater" ("string"), "\r") -> (w2727:string)
                n1819 = Concatenate Strings(w2803, w2802, w2795, w2788, w2781, w2776, w2775, w2768, w2758, w2750, w2729, w2728, w2727, w2726, w2725) -> (w2709:string)
                "gain" <- w2709
              }
              frame #1 {
                n1820 = local read "Camera Port :"() -> (w2817:string)
                n1821 = local read "C3 :"() -> (w2825:refnum<visa-resource-name>)
                n1822 = local read "TEMP INTERCEPT:"() -> (w2826:dbl)
                n1823 = local read "AIR TEMP INTERCEPT:"() -> (w2827:dbl)
                n1824 = local read "Com Port 3"() -> (w2828:refnum<visa-resource-name>)
                n1825 = Concatenate Strings("[CH8]" ("string"), w2817, "- Visa Camera" ("string"), "\r") -> (w2816:string)
                n1826 = Concatenate Strings("[CH7]" ("string"), w2825, "- Visa Humidity" ("string"), "\r") -> (w2821:string)
                n1827 = Number To Fractional String(number=w2826, width (-)=i16 10 ("precision (6)"), precision (6)=i16 5) -> (F-format string=w2844:string)  [unwired: 1 in]
                n1828 = Concatenate Strings("[CHL]" ("string"), w2828, "- Visa humid" ("string"), "\r") -> (w2831:string)
                n1829 = Number To Fractional String(number=w2827, width (-)=i16 10 ("precision (6)"), precision (6)=i16 5) -> (F-format string=w2851:string)  [unwired: 1 in]
                n1830 = Concatenate Strings("[CHK]" ("string"), w2844, "-TEMP INTERCEPT" ("string"), "\r") -> (w2840:string)
                n1831 = Concatenate Strings("[SNO]" ("string"), "S.NO", "-" ("string"), "\r") -> (w2836:string)
                n1832 = Concatenate Strings("[CHJ]" ("string"), w2851, "-AIR TEMP INTERCEPT" ("string"), "\r") -> (w2841:string)
                n1833 = String To Path(string="C:\\LAB-IQ\\calibrate WO 2465.dcf") -> (path=w2829:path)
                n1834 = Concatenate Strings(w2856, w2841, w2840, w2836, w2831, w2821, w2816) -> (w2855:string)
                n1835 = call <vilib>:"Write Characters To File.vi"("append to file? (new file:F)"=FALSE, "character string"=w2855, "file path (dialog if empty)"=w2829) -> ()  [unwired: 2 in, 1 out]
              }
              frame #2 {
                n1836 = local write "Lan flag"(0.0 ("Lan flag")) -> ()
                n1837 = local write "conststatus"(0.0 ("rpm value : 2")) -> ()
                n1838 = local write "SAVE"(FALSE ("OK Button 14")) -> ()
                n1839 = local write "SAVE 2"(FALSE ("SAVE 2")) -> ()
              }
            }
          }
        }
        n1840 = Subtract(x=w2501, y=w2500) -> (x-y=w2502:dbl)
        n1841 = local read "AIR TEMPERATURE : 2"() -> (w2505:dbl)
        n1842 = local read "AIR TEMPERATURE :"() -> (w2504:dbl)
        n1843 = Divide(x=w2502, y=w2500) -> (x/y=w2524:dbl)
        n1844 = Subtract(x=w2517, y=w2516) -> (x-y=w2515:dbl)
        n1845 = Subtract(x=w2508, y=w2506) -> (x-y=w2507:dbl)
        n1846 = Subtract(x=w2514, y=w2513) -> (x-y=w2512:dbl)
        n1847 = Subtract(x=w2510, y=w2509) -> (x-y=w2511:dbl)
        n1848 = Subtract(x=w2505, y=w2504) -> (x-y=w2503:dbl)
        n1849 = Divide(x=w2515, y=w2516) -> (x/y=w2535:dbl)
        n1850 = Divide(x=w2507, y=w2506) -> (x/y=w2528:dbl)
        n1851 = Divide(x=w2512, y=w2513) -> (x/y=w2532:dbl)
        n1852 = Divide(x=w2511, y=w2509) -> (x/y=w2531:dbl)
        n1853 = Multiply(x=w2524, y=100.0) -> (x*y=→"HUMIDITY  Calibration Error":dbl)
        n1854 = Divide(x=w2503, y=w2504) -> (x/y=w2527:dbl)
        n1855 = Multiply(x=w2535, y=100.0) -> (x*y=→"FRIC. FORCE Calibration Error":dbl)
        n1856 = Multiply(x=w2528, y=100.0) -> (x*y=→"TEMPERATURE  Calibration Error":dbl)
        n1857 = Multiply(x=w2532, y=100.0) -> (x*y=→"STROKE Calibration Error":dbl)
        n1858 = Multiply(x=w2531, y=100.0) -> (x*y=→"DISPLACEMENT  Calibration Error":dbl)
        n1859 = property on="EDIT 2" class="Bool (strict)"("Visible"=w2495) -> ()  [unwired: 2 in, 2 out]
        n1860 = property on="SAVE" class="Bool (strict)"("Visible"=w2495) -> ()  [unwired: 2 in, 2 out]
        n1861 = property on="SrvM CP" class="Bool (strict)"("Disabled"=w2496) -> ()  [unwired: 2 in, 2 out]
        n1862 = property on="visa due" class="CmbBox"("Disabled"=w2496) -> ()  [unwired: 2 in, 2 out]
        n1863 = property on="File Path" class="Path"("Disabled"=w2496) -> ()  [unwired: 2 in, 2 out]
        n1864 = Multiply(x=w2527, y=100.0) -> (x*y=→"AIR TEMPERATURE  Calibration Error":dbl)
        n1865 = property on="Language Selection" class="Enum (strict)"("Visible"=w2495) -> ()  [unwired: 2 in, 2 out]
        n1866 = property on="Tab Control 7" class="TabCtl (strict)"("Disabled"=w2496) -> ()  [unwired: 2 in, 2 out]
        n1867 = property on="AIR TEMP INTERCEPT:" class="DigNum (strict)"("Disabled"=w2496) -> ()  [unwired: 2 in, 2 out]
        n1868 = property on="CH-POWER -" class="DigNum (strict)"("Disabled"=w2496) -> ()  [unwired: 2 in, 2 out]
        n1869 = property on="CH-POWER +" class="DigNum (strict)"("Disabled"=w2496) -> ()  [unwired: 2 in, 2 out]
        n1870 = property on="AIR TEMPERATURE :" class="DigNum (strict)"("Disabled"=w2496) -> ()  [unwired: 2 in, 2 out]
        n1871 = property on="STROKE GAIN :" class="DigNum (strict)"("Disabled"=w2496) -> ()  [unwired: 2 in, 2 out]
        n1872 = property on="SPEED OUT:" class="DigNum (strict)"("Disabled"=w2496) -> ()  [unwired: 2 in, 2 out]
        n1873 = property on="CH-HUMIDITY DRY" class="DigNum (strict)"("Disabled"=w2496) -> ()  [unwired: 2 in, 2 out]
        n1874 = property on="HUMIDITY:" class="DigNum (strict)"("Disabled"=w2496) -> ()  [unwired: 2 in, 2 out]
        n1875 = property on="CH-HUMIDITY WET" class="DigNum (strict)"("Disabled"=w2496) -> ()  [unwired: 2 in, 2 out]
        n1876 = property on="TEMPERATURE :" class="DigNum (strict)"("Disabled"=w2496) -> ()  [unwired: 2 in, 2 out]
        n1877 = property on="DISPLACEMENT :" class="DigNum (strict)"("Disabled"=w2496) -> ()  [unwired: 2 in, 2 out]
        n1878 = property on="CH-HEATER" class="DigNum (strict)"("Disabled"=w2496) -> ()  [unwired: 2 in, 2 out]
        n1879 = property on="TEMP INTERCEPT:" class="DigNum (strict)"("Disabled"=w2496) -> ()  [unwired: 2 in, 2 out]
        n1880 = property on="FRIC. FORCE :" class="DigNum (strict)"("Disabled"=w2496) -> ()  [unwired: 2 in, 2 out]
      }
    }
    n1881 = local read "RUN"() -> (w1890:bool)
    n1882 = local read "RUN"() -> (w1888:bool)
    n1883 = disable-structure shown="Disabled" {
      disable-tunnel: [w1905 _] -> w1871
      disable-tunnel: [w1904 _] -> w1869
      frame Disabled {
        n1884 = local read "Temperature before test"() -> (w1898:dbl)
        n1885 = local read "Temperature after test"() -> (w1911:dbl)
        n1886 = case shown="True" "Save Results" {
          frame False {
          }
          frame True {
            w1927 = "\r"
            n1887 = local write "Save Results"(FALSE ("OK Button 5")) -> ()
            n1888 = local read "Temperature before test"() -> (w1965:dbl)
            n1889 = local read "Temperature after test"() -> (w1967:dbl)
            n1890 = local read "Humidity before test"() -> (w1964:dbl)
            n1891 = local read "Humidity after test"() -> (w1966:dbl)
            n1892 = local read "WS1.4"() -> (w1971:dbl)
            n1893 = local read "AVP"() -> (w1969:dbl)
            n1894 = Number To Fractional String(number=w1971, width (-)=i16 6, precision (6)=i16 1) -> (F-format string=w1931:string)  [unwired: 1 in]
            n1895 = local read "MWSD"() -> (w1968:dbl)
            n1896 = local read "String"() -> (w1960:string)
            n1897 = local read "FILE"() -> (w1963:string)
            n1898 = local read "HCF"() -> (w1970:dbl)
            n1899 = Number To Fractional String(number=w1964, width (-)=i16 6, precision (6)=i16 1) -> (F-format string=w1956:string)  [unwired: 1 in]
            n1900 = Number To Fractional String(number=w1965, width (-)=i16 6, precision (6)=i16 1) -> (F-format string=w1953:string)  [unwired: 1 in]
            n1901 = Number To Fractional String(number=w1966, width (-)=i16 6, precision (6)=i16 1) -> (F-format string=w1949:string)  [unwired: 1 in]
            n1902 = Number To Fractional String(number=w1967, width (-)=i16 6, precision (6)=i16 1) -> (F-format string=w1945:string)  [unwired: 1 in]
            n1903 = Number To Fractional String(number=w1969, width (-)=i16 6, precision (6)=i16 3) -> (F-format string=w1938:string)  [unwired: 1 in]
            n1904 = Concatenate Strings(w1960, w1963) -> (w1982:string)
            n1905 = Number To Fractional String(number=w1968, width (-)=i16 6, precision (6)=i16 1) -> (F-format string=w1942:string)  [unwired: 1 in]
            n1906 = Number To Fractional String(number=w1970, width (-)=i16 6, precision (6)=i16 2) -> (F-format string=w1936:string)  [unwired: 1 in]
            n1907 = Concatenate Strings("(" ("string"), w1931, ")Microns" ("string")) -> (w1930:string)
            n1908 = local read "REMARKS"() -> (w1962:string)
            "REMARKS 2" <- w1962
            n1909 = Concatenate Strings("(" ("string"), w1956, " ) % RH," ("string")) -> (w1957:string)
            n1910 = Concatenate Strings(w1936, ")" ("string")) -> (w1934:string)
            n1911 = Concatenate Strings("(" ("string"), w1953, ")  Deg C ," ("string")) -> (w1952:string)
            n1912 = Concatenate Strings("(" ("string"), w1949, " ) % RH," ("string")) -> (w1948:string)
            n1913 = Concatenate Strings("(" ("string"), w1945, ")  Deg C ," ("string")) -> (w1944:string)
            n1914 = Concatenate Strings("(" ("string"), w1942, ")  Microns," ("string")) -> (w1941:string)
            n1915 = Concatenate Strings("(" ("string"), w1938, ")  kPa," ("string")) -> (w1928:string)
            n1916 = Concatenate Strings(w1982, ".dwm" ("Substring")) -> (w1980:string)
            n1917 = String To Path(string=w1980) -> (path=w1979:path)
            n1918 = Concatenate Strings(w1962, w1927, " Humidity before test= " ("Substring"), w1957, w1927, " Temperature before test = " ("Substring"), w1952, w1927, " Humidity after test= " ("Substring"), w1948, w1927, "Temperature after test = " ("Substring"), w1944, w1927, "MSD = " ("Substring"), w1941, w1927, "  AVP = " ("Substring"), w1928, w1927, "  HCF                     =( " ("Substring"), w1934, w1927, " WS1.4                  = " ("Substring"), w1930, w1927) -> (w1926:string)
            "data" <- w1926
            n1919 = call <vilib>:"Write Characters To File.vi"("append to file? (new file:F)"=FALSE, "character string"=w1926, "file path (dialog if empty)"=w1979) -> ()  [unwired: 2 in, 1 out]
            n1920 = Match Pattern(string=w1926, regular expression="!") -> (after substring=→"export":string)  [unwired: 1 in, 3 out]
          }
        }
        n1921 = Add(x=231.864, y=w1898) -> (x+y=w1895:dbl)
        n1922 = Add(x=231.864, y=w1911) -> (x+y=w1908:dbl)
        n1923 = Divide(x=1705.984, y=w1895) -> (x/y=w1896:dbl)
        n1924 = Divide(x=1705.984, y=w1908) -> (x/y=w1909:dbl)
        n1925 = local read "Humidity before test"() -> (w1900:dbl)
        n1926 = local read "Humidity after test"() -> (w1913:dbl)
        n1927 = Subtract(x=8.017352 ("y"), y=w1896) -> (x-y=w1922:dbl)
        n1928 = Subtract(x=8.017352 ("y"), y=w1909) -> (x-y=w1916:dbl)
        n1929 = expression code="10**y"(w1922) -> (w1902:dbl)
        n1930 = expression code="10**y"(w1916) -> (w1915:dbl)
        n1931 = Multiply(x=w1900, y=w1902) -> (x*y=w1901:dbl)
        n1932 = Multiply(x=w1913, y=w1915) -> (x*y=w1914:dbl)
        n1933 = Divide(x=w1901, y=750.0) -> (x/y=w1917:dbl)
        n1934 = Divide(x=w1914, y=750.0) -> (x/y=w1918:dbl)
        n1935 = Add(x=w1917, y=w1918) -> (x+y=w1919:dbl)
        n1936 = Divide(x=w1919, y=2.0) -> (x/y=w1921:dbl)
        n1937 = local write "AVP"(w1921) -> ()
        n1938 = Subtract(x=1.4, y=w1921) -> (x-y=w1904:dbl)
        n1939 = local read "HCF"() -> (w1905:dbl)
      }
      frame Enabled {
      }
    }
    n1940 = case shown="True" "EDIT 3" {
      frame False {
      }
      frame True {
        n1941 = local write "EDIT 3"(FALSE ("EDIT 3")) -> ()
        n1942 = local write "Main Tab"(T2."About" ("Main Tab")) -> ()
      }
    }
    n1943 = case shown="False" w1890 {
      frame False {
        n1944 = local read "stopT"() -> (w2868:bool)
        n1945 = case shown="True" w2868 {
          frame False {
          }
          frame True {
            n1946 = local write "stopT"(FALSE) -> ()
          }
        }
      }
      frame True {
        "stopT" <- TRUE
      }
    }
    n1947 = case shown="False" w1888 {
      frame False {
      }
      frame True {
      }
    }
    n1948 = case shown="True" w1878 {
      frame False {
        n1949 = property on="Password 2" class="Str"("Visible"=FALSE) -> ()  [unwired: 2 in, 2 out]
        n1950 = local write "Password 2"("" ("Password")) -> ()
      }
      frame True {
        n1951 = property on="Password 2" class="Str"("Visible"=TRUE) -> ()  [unwired: 2 in, 2 out]
        n1952 = Equal?(x="Password 2", y="HFRR1234") -> (x = y?=w2010:bool)
        n1953 = case shown="True" w2010 {
          tunnel: "Password 2" -> [w2013 _]
          frame False {
            n1954 = String Length(string=w2013) -> (length=w2014:i32)
            n1955 = Greater Than 0?(x=w2014) -> (x > 0?=w2012:bool)
            n1956 = case shown="False" w2012 {
              frame False {
                n1957 = property on="Password 2" class="Str"("Caption.Text"="Password (Advance Setting)") -> ()  [unwired: 2 in, 2 out]
              }
              frame True {
                n1958 = property on="Password 2" class="Str"("Caption.Text"="Incorrect Password!") -> ()  [unwired: 2 in, 2 out]
              }
            }
          }
          frame True {
            n1959 = local write "EDIT 2"(FALSE ("EDIT 2")) -> ()
            n1960 = local write "Password 2"("" ("Password")) -> ()
            n1961 = local write "Main Tab"(T2."Advance" ("Main Tab")) -> ()
            n1962 = local write "Main Dashboard Buttons"(T1."Advance" ("Main Dashboard Buttons")) -> ()
          }
        }
      }
    }
    n1963 = case shown="True" "Prog Uno" {
      frame False {
      }
      frame True {
        n1964 = stacked-sequence {
          frame #0 {
            n1965 = Delete(path (use dialog)=path "C:/LAB-IQ-NXT/UNOCOMPILE.bat" ("working directory")) -> ()  [unwired: 4 in, 3 out]
          }
          frame #1 {
            n1966 = local read "Com Port 1"() -> (w2475:refnum<visa-resource-name>)
            n1967 = Concatenate Strings("cmd.exe /c \"mode " ("command line"), w2475, ":1200,n,8,1\"\n" ("command line")) -> (w2480:string)
            n1968 = Concatenate Strings(w2480, "CD\\\nCD WinDucom\navrdude -C avrdude.conf -v -patmega328p -carduino -P" ("command line"), w2475, " -b115200 -D -Uflash:w:UNO_V20.hex:i\n" ("command line"), "\r") -> (w2482:string)
            "STR" <- w2482
            n1969 = call <vilib>:"Write Characters To File.vi"("append to file? (new file:F)"=FALSE, "character string"=w2482, "file path (dialog if empty)"=path "C:/LAB-IQ/UNOCOMPILE.bat" ("working directory")) -> ()  [unwired: 2 in, 1 out]
          }
          frame #2 {
            n1970 = disable-structure shown="Disabled" {
              frame Disabled {
                w2486 = "cmd.exe  /c \"C:\\LAB-IQ-NXT\\UNOCOMPILE.bat\"" ("string")
                n1971 = local write "Prog Uno"(FALSE ("run minimized? (F)")) -> ()
                n1972 = call <vilib>:"System Exec.vi"("expected output size  (4096)"=u32 65535, "run minimized? (F)"=FALSE, "wait until completion? (T)"=TRUE ("run minimized? (F)"), "working directory"=path "C:/LAB-IQ-NXT", "standard input"=w2486, "command line"=w2486) -> ("error out"=w2485:errorcluster, "standard output"=→"String 42":string)  [unwired: 2 in, 2 out]
                "error out 3" <- w2485
                n1973 = flat-sequence {
                  tunnel: w2485 -> [_]
                  frame #0 {
                  }
                }
              }
              frame Enabled {
              }
            }
          }
        }
      }
    }
    n1974 = case shown="\"ISO 12156\"" "TEST STANDARD" {
      tunnel: [2.0 ("Set Temp") 0.0 ("Set Temp") 2.0 ("Set Temp") 0.0 ("Set Temp")] -> w1879
      frame "ASTM D6079", Default {
        w2432 = 50.0 ("Hz")
        w2433 = 53.0 ("Set Rh")
        w2435 = 1.0 ("Set Strk")
        w2434 = 60.0 ("Set Temp")
        # "astm hide"
        n1975 = local write "NORMAL LOAD"(200.0 ("NORMAL LOAD")) -> ()
        n1976 = local write "Set Strk"(w2435) -> ()
        n1977 = local write "Set Hz"(w2432) -> ()
        n1978 = local write "Set Temp"(w2434) -> ()
        n1979 = local write "Set Rh"(w2433) -> ()
        n1980 = local write "test time"(75.0 ("test time")) -> ()
        n1981 = local write "Set Stroke:"(w2435) -> ()
        n1982 = local write "Set Humidity:"(w2433) -> ()
        n1983 = local write "Set Frequency:"(w2432) -> ()
        n1984 = local write "Set Temperature:"(w2434) -> ()
        "Test Standard" <- "ASTM D6079" ("Test Standard 2")
      }
      frame "ISO 12156" {
        n1985 = local write "Set Strk"(1.0 ("Set Strk")) -> ()
        n1986 = local write "NORMAL LOAD"(200.0 ("NORMAL LOAD")) -> ()
        n1987 = local write "Set Temp"(60.0 ("Set Temp")) -> ()
        n1988 = local write "test time"(75.0 ("test time")) -> ()
        n1989 = local write "Set Hz"(50.0 ("Hz")) -> ()
        n1990 = local write "Set Rh"(53.0 ("Set Rh")) -> ()
      }
      frame "CEC F-096-A-06" {
        n1991 = local write "Set Strk"(1.0 ("Set Strk")) -> ()
        n1992 = local write "NORMAL LOAD"(200.0 ("NORMAL LOAD")) -> ()
        n1993 = local write "Set Temp"(60.0 ("Set Temp")) -> ()
        n1994 = local write "test time"(75.0 ("test time")) -> ()
        n1995 = local write "Set Hz"(50.0 ("Hz")) -> ()
        n1996 = local write "Set Rh"(53.0 ("Set Rh")) -> ()
      }
      frame "Custom" {
      }
    }
    n1997 = case shown="True" "Prog Due" {
      frame False {
      }
      frame True {
        n1998 = stacked-sequence {
          frame #0 {
            n1999 = Delete(path (use dialog)=path "C:/LAB-IQ/DUECOMPILE.bat" ("working directory")) -> ()  [unwired: 4 in, 3 out]
          }
          frame #1 {
            n2000 = disable-structure shown="Disabled" {
              frame Disabled {
                n2001 = local read "visa due"() -> (w2457:string)
                n2002 = Concatenate Strings("cmd.exe /c \"mode " ("command line"), w2457, ":1200,n,8,1\"\n" ("command line")) -> (w2462:string)
                n2003 = Concatenate Strings(w2462, "CD\\\nCD WinDucom\nTIMEOUT 1\n bossac.exe -i -d --port=" ("command line"), w2457, " -U false -e -w -v -b DUE.bin -R\n" ("command line"), "\r") -> (w2464:string)
                "concatenated string 2" <- w2464
                n2004 = call <vilib>:"Write Characters To File.vi"("append to file? (new file:F)"=FALSE, "character string"=w2464, "file path (dialog if empty)"=path "C:/LAB-IQ-NXT/DUECOMPILE.bat" ("working directory")) -> ()  [unwired: 2 in, 1 out]
              }
              frame Enabled {
              }
            }
          }
          frame #2 {
            # "C:\\LAB-IQ-NXT\\DUECOMPILE.bat"
            n2005 = disable-structure shown="Disabled" {
              frame Disabled {
                w2469 = "cmd.exe  /c \"C:\\LAB-IQ-NXT\\DUECOMPILE.bat\"" ("string")
                n2006 = call <vilib>:"System Exec.vi"("expected output size  (4096)"=u32 65535, "run minimized? (F)"=FALSE, "wait until completion? (T)"=TRUE ("run minimized? (F)"), "working directory"=path "C:/LAB-IQ-NXT", "standard input"=w2469, "command line"=w2469) -> ("error out"=w2468:errorcluster, "standard output"=→"String 44":string)  [unwired: 2 in, 2 out]
                "error out 4" <- w2468
                n2007 = flat-sequence {
                  tunnel: w2468 -> [_]
                  frame #0 {
                  }
                }
              }
              frame Enabled {
              }
            }
            n2008 = local write "Prog Due"(FALSE ("Prog Due")) -> ()
          }
        }
      }
    }
    n2009 = Or(x=w1876, y=w1874) -> (x .or. y?=w1875:bool)
    n2010 = case shown="\"About\"" w1873 {
      tunnel: [T27."Acquire" ("Main Tab") T27."Compare Files" ("Main Tab") T27."About" ("Main Tab")] -> w1886
      frame "Acquire", Default {
      }
      frame "Compare Files" {
      }
      frame "About" {
      }
    }
    n2011 = Or(x=w1880, y="OPEN") -> (x .or. y?=w1881:bool)
    n2012 = case shown="True" w1881 {
